vi "CThread Cancel.vi"   [LabVIEW 2012, in "CThread.lvlib"]
uses:
  CThread.lvlib
  XNodes/terminalnode/CThread VI Terminal Node.xnode
  Base/CThread Base - Cancel.vi
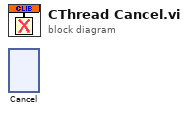
[diagram p0: block diagram]
diagram:
  n1 = xnode "Cancel"() -> ()  [unwired: 1 in, 1 out]
